vi "creatdvice.vi"(3 "数值":i32) -> (0 "ddrlength":i32, 1 "hDevice":i32)   [LabVIEW 2012]
panel:
  out "ulDDR2Length":i32
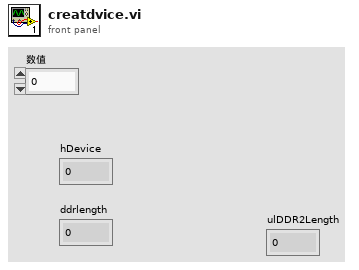
[diagram p1: front panel]
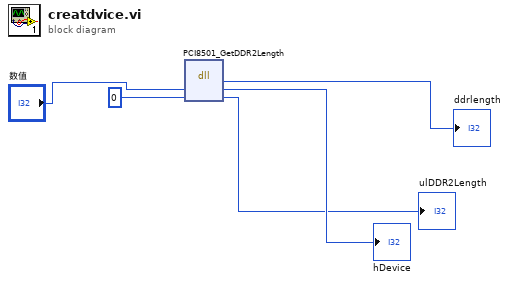
[diagram p0: block diagram]
diagram:
  n1 = dll-call lib="PCI8501_32" fn="PCI8501_GetDDR2Length" label="GetDDR2Length"("hDevice"="数值", "ulDDR2Length"=0) -> ("返回类型"=→"ddrlength":i32, "hDevice"=→"hDevice":i32, "ulDDR2Length"=→"ulDDR2Length":i32)  [unwired: 3 in, 2 out]
